vi "SMU.Keithley2600.SetResource.vi"(8 "error in (no error)":errorcluster, 10 "Resource":T1, 11 "SMU.Keithley2600 in":refnum<class "SMU.Keithley2600.lvclass">) -> (0 "error out":errorcluster, 3 "SMU.Keithley2600 out":refnum<class "SMU.Keithley2600.lvclass">)   [LabVIEW 2017, in "SMU.Keithley2600.lvclass"]
uses:
  SMU.Keithley2600.lvclass
  Typedefs/Resource--Cluster.ctl
  <instrlib>/Keithley 2600 Series/Public/Channel.ctl
  SMU.Keithley2600.lvclass/SMU.Keithley2600.ctl
  <instrlib>/Keithley 2600 Series/Keithley 2600 Series.lvlib
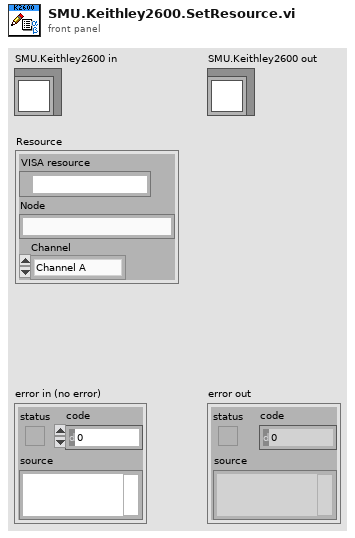
[diagram p1: front panel]
types:
  T1 = typedef "SMU.Keithley2600.lvclass/Resource--Cluster.ctl" = cluster{"VISA resource":refnum<visa-resource-name>, "Node":string, "Channel":T2}
  T2 = typedef "Keithley 2600 Series.lvlib/Channel.ctl" = enum32{"Channel A", "Channel B"}
  T3 = typedef "SMU.Keithley2600.lvclass/PrivateData--Ref.ctl" = refnum<data-value>
  T4 = typedef "SMU.Keithley2600.lvclass/PrivateData--Cluster.ctl" = cluster{"Resource":T1}
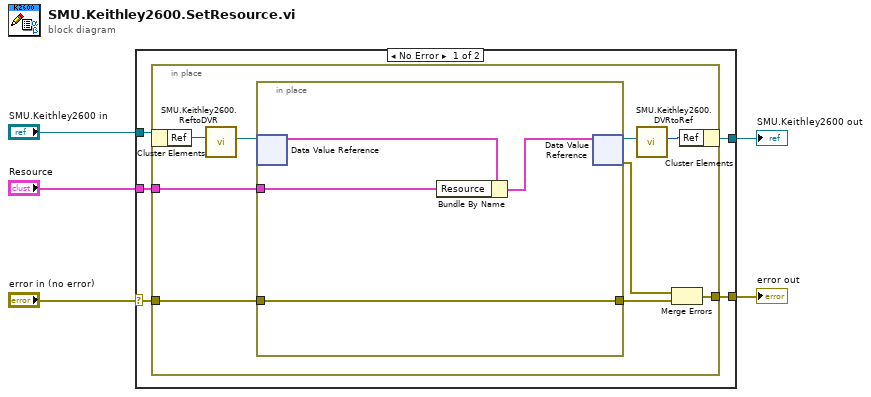
[diagram p0: block diagram]
diagram:
  n1 = case shown="No Error" "error in (no error)" {
    selector: "error in (no error)" -> [w8 w25]
    tunnel: [w9 w25] -> w4
    tunnel: [w7 w24] -> w2
    tunnel: "SMU.Keithley2600 in" -> [w10 w24]
    tunnel: "Resource" -> [w6 _]
    frame No Error {
      n2 = in-place {
        in-place-border: [w16] -> w9
        in-place-border: w8 -> [w14]
        in-place-border: w6 -> [w11]
        n3 = in-place-cluster #1(w10) -> ("Ref"=w18:u32)
        n4 = call "SMU.Keithley2600.ReftoDVR.vi"("Ref"=w18) -> ("Ref"=w17:T3)  [unwired: 10 in]
        n5 = in-place {
          in-place-border: w14 -> [w21]
          in-place-border: [w21] -> w13
          in-place-border: w11 -> [w20]
          n6 = in-place-dvr #2(w17) -> (w23:T4)  [unwired: 1 out]
          n7 = Bundle By Name(cluster=w23, "Resource"=w20) -> (w22:T4)
          n8 = in-place-dvr #2(w22) -> (w12:T3, w15:errorcluster)
        }
        n9 = call "SMU.Keithley2600.DVRtoRef.vi"("Ref"=w12) -> ("Ref"=w19:u32)  [unwired: 10 in]
        n10 = Merge Errors(w15, w13) -> (w16:errorcluster)
        n11 = in-place-cluster #1("Ref"=w19) -> (w7:refnum<class "SMU.Keithley2600.lvclass">)
      }
    }
    frame Error {
    }
  }
  "error out" <- w4
  "SMU.Keithley2600 out" <- w2
